vi "SubConfocal_Initialize.vi"(8 "error in":errorcluster, 11 "VISA  IN":refnum<visa-resource-name>="COM1") -> (0 "error out":errorcluster, 3 "VISA OUT":refnum<visa-resource-name>="COM1")   [LabVIEW 2015]
doc: "VI initializes and configues the MAC5000; the user chooses whether communication with the MAC5000 occurs over the Serial Port(RS232) or the USB port. This VI should be run once at the beginning of a larger program.\n\nNote: \nSerial Port communication occurs over Serial Port 1; if the user wants to use a different Serial Port the VISA Resource name needs to be changed in the block diagram from ASRL1::INSTR to ASRL#::INSTR where # is the number of the Serial Port.\nTo use USB communication, the user needs to set up the VISA protocol using the VISA driver development wizard. After setting up the VISA driver, the user needs to enter the correct VISA resource name in the block diagram. Note the VISA resource name is specific to a particular USB Bus; if the MAC5000 is plugged into another USB bus the user needs to set up the VISA resource name again."
uses:
  <vilib>/Instr/_visa.llb/VISA Configure Serial Port (Instr).vi
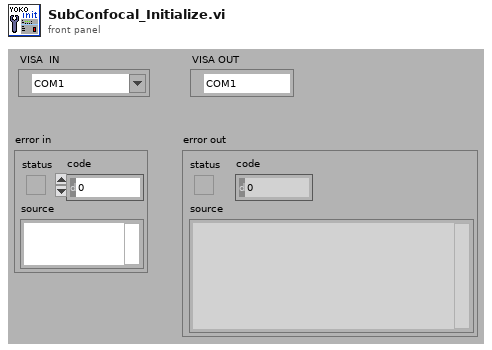
[diagram p1: front panel]
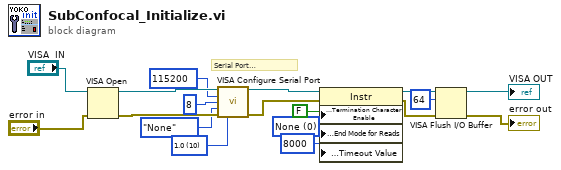
[diagram p0: block diagram]
diagram:
  w1 = u16 10 items=["1.0"=10, "1.5"=15, "2.0"=20] ("stop bits (10: 1 bit)")
  w8 = u16 0 items=["None", "LastBit", "TermChar"] ("Serial Settings:Serial End Mode for Reads")
  # "Serial Port Configuration"
  n1 = VISA Open(error in (no error)="error in", VISA resource name="VISA  IN") -> (VISA resource name=w17:refnum<visa-resource-name>, error out=w16:errorcluster)  [unwired: 3 in]
  n2 = call-poly "VISA Configure Serial Port"("VISA resource name"=w17, "baud rate (9600)"=u32 115200, "data bits (8)"=u16 8, "parity (0:none)"=enum16{"None", "Odd", "Even", "Mark", "Space"}."None", "error in (no error)"=w16, "stop bits (10: 1 bit)"=w1) -> ("VISA resource name out"=w6:refnum<visa-resource-name>, "error out"=w5:errorcluster)  [unwired: 8 in]
  n3 = property class="Instr"(reference=w6, error in=w5, "Message Based Settings:Termination Character Enable"=FALSE, "Serial Settings:End Mode for Reads"=w8, "General Settings:Timeout Value"=u32 8000) -> (reference out=w3:refnum<visa-resource-name>, error out=w2:errorcluster)
  n4 = VISA Flush I/O Buffer(VISA resource name=w3, mask (16)=u16 64, error in (no error)=w2) -> (VISA resource name out=→"VISA OUT":refnum<visa-resource-name>, error out=→"error out":errorcluster)
